vi "Temperature Grad Read Single.vi"(8 "error in":errorcluster, 9 "Channel Index":i32=1, 11 "Chiller in":refnum<class "Chiller.lvclass">) -> (0 "error out":errorcluster, 1 "Changed or First Call?":bool, 2 "Temperature SP":dbl, 3 "Chiller out":refnum<class "Chiller.lvclass">)   [LabVIEW 2023, in "Chiller.lvclass"]
uses:
  Chiller.lvclass
  Chiller.lvclass/Chiller.ctl
  Low Level Capabilities/Temperature/Temperature Gradient/Temperature Gradient.lvclass
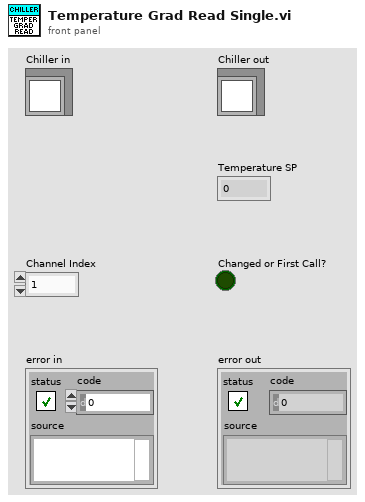
[diagram p1: front panel]
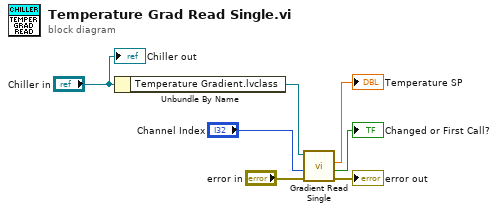
[diagram p0: block diagram]
diagram:
  n1 = Unbundle By Name("Chiller in") -> ("Temperature Gradient.lvclass"=w7:refnum<class "Temperature Gradient.lvclass">)
  n2 = call-dynamic "Gradient Read Single.vi"("error in"="error in", "Channel Index"="Channel Index", "Temperature Gradient in"=w7) -> ("error out"=→"error out":errorcluster, "Changed or First Call?"=→"Changed or First Call?":bool, "Temperature SP"=→"Temperature SP":dbl)  [unwired: 5 in, 1 out]
  "Chiller out" <- "Chiller in"
